vi "Configure Current and Voltage.vi"(0 "VISA session":refnum<visa-resource-name>, 5 "V Range (12: 1000)":u16(ring)=12 items=["AUTO", "1.5", "3", "6", "10", "15", "30", "60", "100", "150", "300", "600", "1000"], 7 "Element (0: All)":u16(ring) items=["All", "Element 1", "Element 2", "Element 3", "Element 4", "Element 5", "Element 6"], 9 "A Range (9: 5A)":u16(ring)=9 items=["AUTO", "10 mA", "20 mA", "50 mA", "100 mA", "200 mA", "500 mA", "1 A", "2 A", "5 A", "10 A", "20 A", "50 A", "S-AUTO", "50 mV", "100 mV", "250 mV", "500 mV", "1 V", "2.5 V", "5 V", "10 V"], 11 "error in (no error)":errorcluster) -> (4 "dup VISA session":refnum<visa-resource-name>, 15 "error out":errorcluster)   [LabVIEW 2012, in "Universal Power Meter.lvlib" / "WT1600.lvlib" / "WT1600.lvclass"]
uses:
  WT1600.lvclass
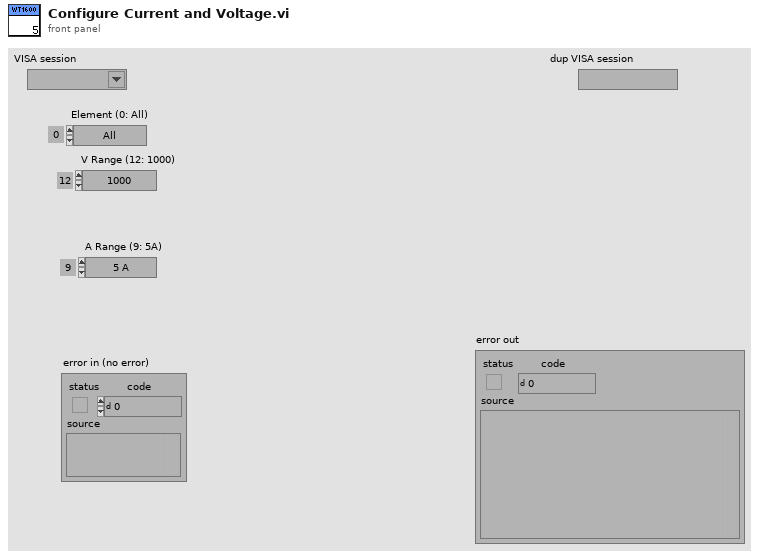
[diagram p1: front panel]
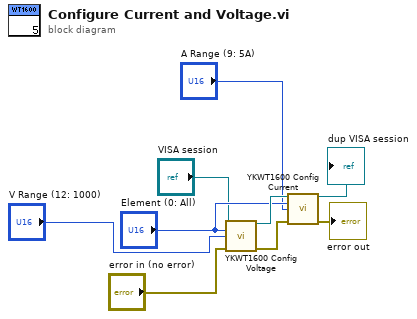
[diagram p0: block diagram]
diagram:
  n1 = call <instrlib>:"YKWT1600 Config Voltage.vi"("VISA session"="VISA session", "Element (0: All)"="Element (0: All)", "V Range (12: 1000)"="V Range (12: 1000)", "error in (no error)"="error in (no error)") -> ("dup VISA session"=w9:refnum<visa-resource-name>, "error out"=w8:errorcluster)  [unwired: 10 in]
  n2 = call <instrlib>:"YKWT1600 Config Current.vi"("VISA session"=w9, "Element (0: All)"="Element (0: All)", "A Range (9: 5A)"="A Range (9: 5A)", "error in (no error)"=w8) -> ("dup VISA session"=→"dup VISA session":refnum<visa-resource-name>, "error out"=→"error out":errorcluster)  [unwired: 10 in]
